vi "Upgrade Addon to Latest Version.vi"(8 "error in (no error)":errorcluster, 11 "Device Item Ref in in":T1 format="%.0x") -> (0 "error out":errorcluster, 3 "Device Item Ref out":T1 format="%.0x")   [LabVIEW 2026, in "FPGA Addon Shared.lvlib"]
uses:
  FPGA Addon Shared.lvlib
  <vilib>/NI VeriStand/Custom Device API/Custom Device Item Ref.ctl
  Types/FG Action.ctl
  Types/Register Information.ctl
  Types/FPGA Addon Data Type.ctl
  <vilib>/rvi/FIFO/Fifo_Types/Fifo_DMA_Config.ctl
  <vilib>/rvi/DataTransferAndStorage/Container/Common/niFpgaDataTypeControl.ctl
  <vilib>/rvi/ClientSDK/Core/ModuleGeneration/CommunicationInterfaceUtility/niFpgaDmaChannelImplementation.ctl
  Types/DMA Information.ctl
  Constants.vi
  <vilib>/NI/NI VeriStand Advanced SysDef API/_SubVIs/SysDef.Search.GUID.vi
  <vilib>/NI/NI VeriStand Advanced SysDef API/_SubVIs/SysDef.Property.Get.Variant.vi
  <vilib>/NI/NI VeriStand Advanced SysDef API/SysDef API/SysDef.Property.Set.vi
  <vilib>/NI/NI VeriStand Advanced SysDef API/_SubVIs/SysDef.Property.Set.Variant.vi
  <vilib>/NI/NI VeriStand Advanced SysDef API/_SubVIs/SysDef.Search.GUIDs.vi
  C:/Users/Administrator/Desktop/Jatin/All DNC DLLs/NationalInstruments.VeriStand.SystemDefinitionAPI.dll
  Jatin/All DNC DLLs/NationalInstruments.VeriStand.SystemDefinitionAPI.dll
  <vilib>/NI/NI VeriStand Advanced SysDef API/SysDef API/Advanced System Definition.lvlib
  <vilib>/NI VeriStand/Custom Device API/Custom Device API.lvlib
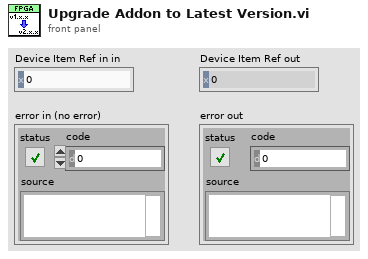
[diagram p1: front panel]
types:
  T1 = typedef "Custom Device API.lvlib/Custom Device Item Ref.ctl" = u64
  T2 = typedef "FPGA Addon Shared.lvlib/FG Action.ctl" = enum8{"GET", "SET"}
  T3 = typedef "FPGA Addon Shared.lvlib/Register Information.ctl" = cluster{"Name":string, "Data Type":T4, "Default Value":variant, "Attributes":variant}
  T4 = typedef "FPGA Addon Shared.lvlib/FPGA Addon Data Type.ctl" = enum8{"<Null>", "I8", "I16", "I32", "I64", "U8", "U16", "U32", "U64", "SGL", "Boolean", "Analog PWM In Settings", "Analog PWM In", "Digital PWM In Settings", "Digital PWM In", "Digital PWM Out", "Sine Out", "FXP", "FXP+/-24.5", "FXP+/-16.5", "FXP+/-32.8", "FXP+/-64.32", "FXP+/-16.7", "FXP+/-20.5", "FXP+/-27.5", "FXP+/-32.16", "FXP+16.3", "FXP+18.3", "Digital Static In", "Digital Static Out", "Digital Static In Settings", "Digital WSS Out", "Quad Encoder Settings", "Quad Encoder In", "Group"}
  T5 = typedef "FPGA Addon Shared.lvlib/DMA Information.ctl" = cluster{"Name":string, "Data Type":T4}
  T6 = cluster{"Name":string, "Data Type":enum8{"<Null>", "I8", "I16", "I32", "I64", "U8", "U16", "U32", "U64", "SGL", "Boolean", "Analog PWM In Settings", "Analog PWM In", "Digital PWM In Settings", "Digital PWM In", "Digital PWM Out", "Sine Out", "FXP+/-24.5", "FXP+/-16.5", "FXP+/-32.8", "FXP+/-64.32", "FXP+/-16.7", "FXP+/-20.5", "FXP+/-27.5", "FXP+/-32.16", "FXP+16.3", "FXP+18.3", "Digital Static In", "Digital Static Out", "Digital Static In Settings", "Digital WSS Out", "Quad Encoder Settings", "Quad Encoder In", "Group"}}[]
  T7 = cluster{"Name":string, "Data Type":enum8{"<Null>", "I8", "I16", "I32", "I64", "U8", "U16", "U32", "U64", "SGL", "Boolean", "Analog PWM In Settings", "Analog PWM In", "Digital PWM In Settings", "Digital PWM In", "Digital PWM Out", "Sine Out", "FXP+/-24.5", "FXP+/-16.5", "FXP+/-32.8", "FXP+/-64.32", "FXP+/-16.7", "FXP+/-20.5", "FXP+/-27.5", "FXP+/-32.16", "FXP+16.3", "FXP+18.3", "Digital Static In", "Digital Static Out", "Digital Static In Settings", "Digital WSS Out", "Quad Encoder Settings", "Quad Encoder In", "Group"}, "Default Value":variant}[]
  T8 = cluster{"Name":string, "Data Type":enum8{"<Null>", "I8", "I16", "I32", "I64", "U8", "U16", "U32", "U64", "SGL", "DBL", "EXT", "CSG", "CDB", "CXT", "0x0F", "0x10", "0x11", "0x12", "0x13", "0x14", "Enum U8", "Enum U16", "Enum U32", "Enum U64", "SGL PQ", "DBL PQ", "EXT PQ", "CSG PQ", "CDB PQ", "CXT PQ", "0x1F", "0x20", "Boolean", "0x22", "0x23", "0x24", "0x25", "0x26", "0x27", "0x28", "0x29", "0x2A", "0x2B", "0x2C", "0x2D", "0x2E", "0x2F", "String", "0x31", "Path", "Pict", "0x34", "0x35", "0x36", "DAQ", "0x38", "0x39", "0x3A", "0x3B", "0x3C", "0x3D", "0x3E", "0x3F", "Array", "0x41", "0x42", "0x43", "0x44", "0x45", "0x46", "0x47", "0x48", "0x49", "0x4A", "0x4B", "0x4C", "0x4D", "0x4E", "0x4F", "Cluster", "0x51", "0x52", "Variant", "Waveform", "0x55", "0x56", "0x57", "0x58", "0x59", "0x5A", "0x5B", "0x5C", "0x5D", "0x5E", "0x5F", "0x60", "0x61", "0x62", "0x63", "0x64", "0x65", "0x66", "0x67", "0x68", "0x69", "0x6A", "0x6B", "0x6C", "0x6D", "0x6E", "0x6F", "Refnum"}, "Default Value":dbl}[]
  T9 = enum8{"<Null>", "I8", "I16", "I32", "I64", "U8", "U16", "U32", "U64", "SGL", "DBL", "EXT", "CSG", "CDB", "CXT", "0x0F", "0x10", "0x11", "0x12", "0x13", "0x14", "Enum U8", "Enum U16", "Enum U32", "Enum U64", "SGL PQ", "DBL PQ", "EXT PQ", "CSG PQ", "CDB PQ", "CXT PQ", "0x1F", "0x20", "Boolean", "0x22", "0x23", "0x24", "0x25", "0x26", "0x27", "0x28", "0x29", "0x2A", "0x2B", "0x2C", "0x2D", "0x2E", "0x2F", "String", "0x31", "Path", "Pict", "0x34", "0x35", "0x36", "DAQ", "0x38", "0x39", "0x3A", "0x3B", "0x3C", "0x3D", "0x3E", "0x3F", "Array", "0x41", "0x42", "0x43", "0x44", "0x45", "0x46", "0x47", "0x48", "0x49", "0x4A", "0x4B", "0x4C", "0x4D", "0x4E", "0x4F", "Cluster", "0x51", "0x52", "Variant", "Waveform", "0x55", "0x56", "0x57", "0x58", "0x59", "0x5A", "0x5B", "0x5C", "0x5D", "0x5E", "0x5F", "0x60", "0x61", "0x62", "0x63", "0x64", "0x65", "0x66", "0x67", "0x68", "0x69", "0x6A", "0x6B", "0x6C", "0x6D", "0x6E", "0x6F", "Refnum"}
  T10 = typedef "Fifo_DMA_Config.ctl" = cluster{"Name":string, "Depth":u32, "Write? (Deprecated:Use Implementation)":bool, "Physical Channel":u32, "Base Address":u32, "Data Width":u32, "Data Type":T11, "FXP Properties":variant, "Write Window Address":u32, "Implementation":T12, "Control Set":u32}
  T11 = typedef "niFpgaDataTypeControl.ctl" = enum32{"Boolean", "I8", "I16", "I32", "I64", "U8", "U16", "U32", "U64", "FXP", "CustomControl", "SGL"}
  T12 = typedef "niFpgaDmaChannelImplementation.ctl" = enum16{"niFpgaTargetToHost", "niFpgaHostToTarget", "niFpgaPeerToPeerWriter", "niFpgaPeerToPeerReader", "niCoreTargetToHost", "niCoreHostToTarget", "niMemoryBufferReader", "niMemoryBufferWriter"}
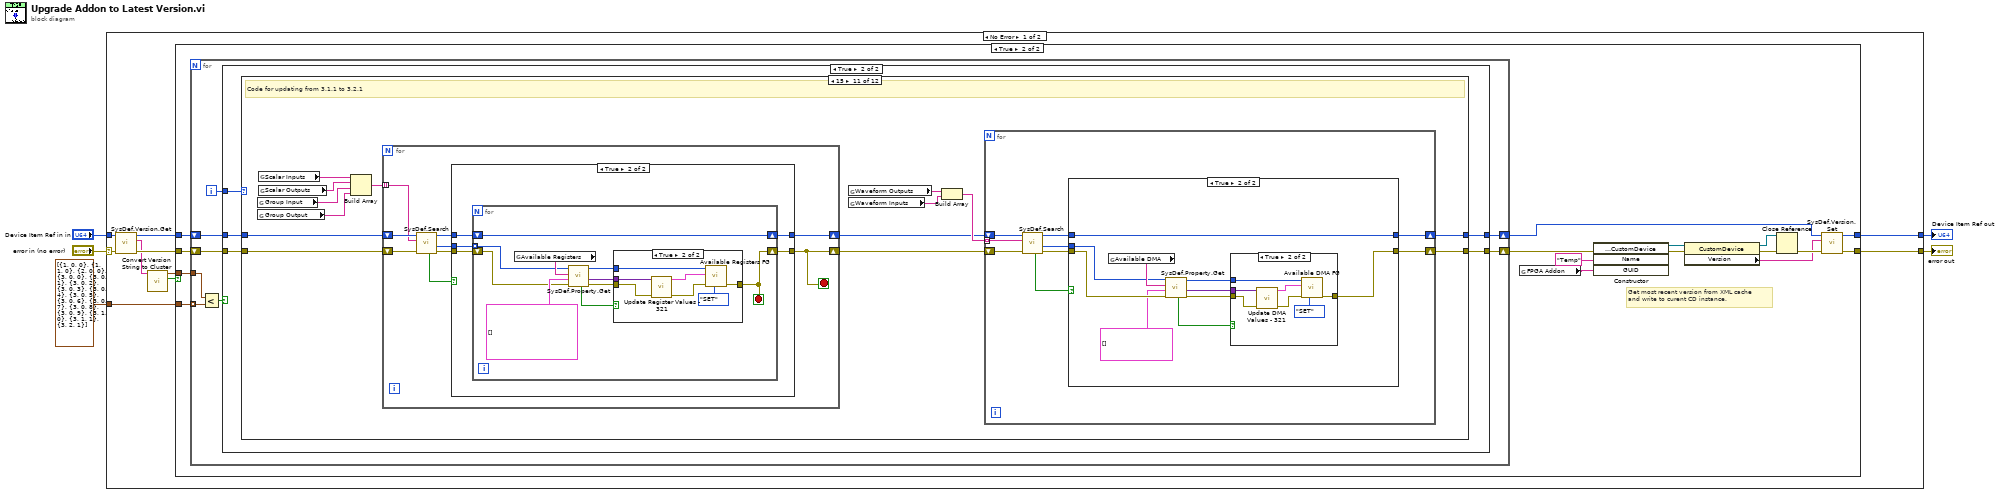
[diagram p0: block diagram]
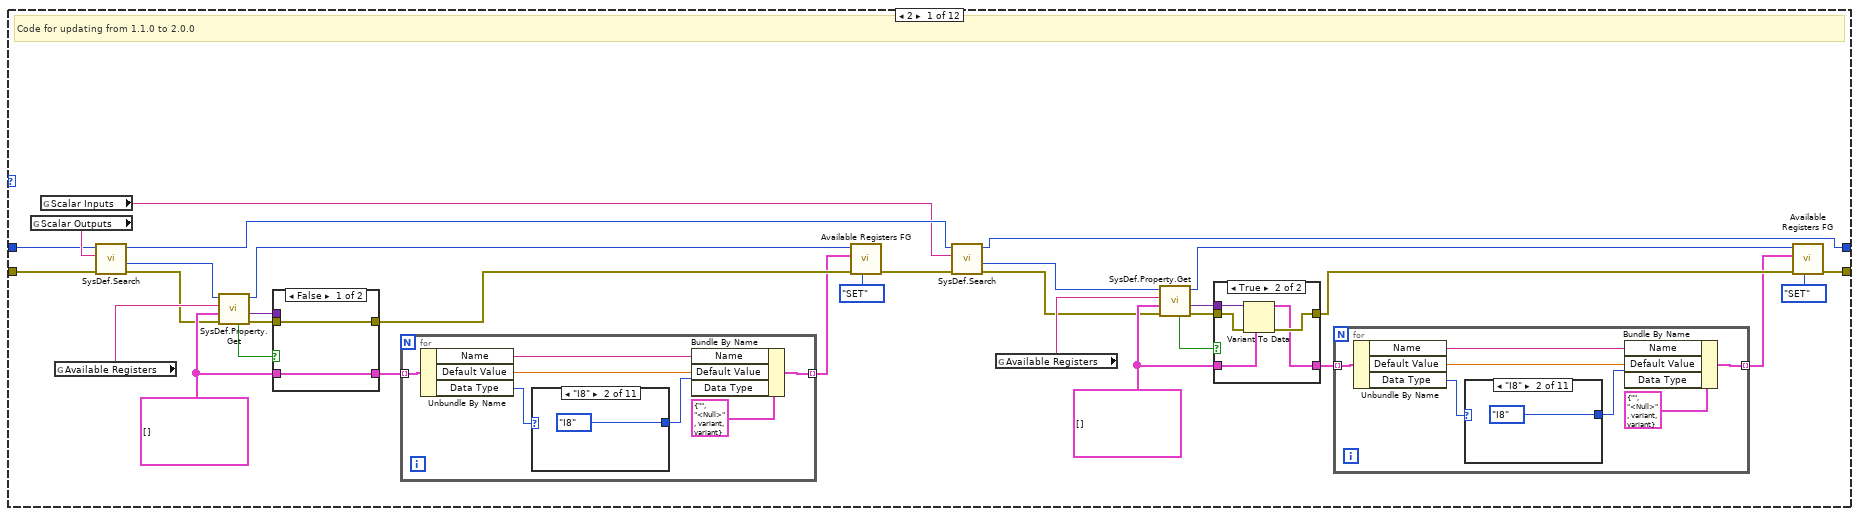
[diagram p4: hidden frame]
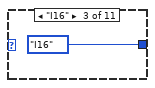
[diagram p6: hidden frame]
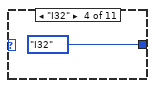
[diagram p7: hidden frame]
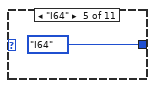
[diagram p8: hidden frame]
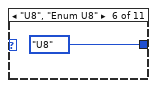
[diagram p9: hidden frame]
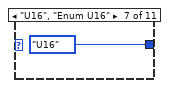
[diagram p10: hidden frame]
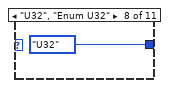
[diagram p11: hidden frame]
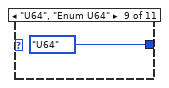
[diagram p12: hidden frame]
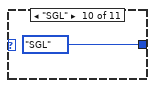
[diagram p13: hidden frame]
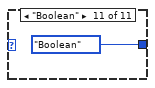
[diagram p14: hidden frame]
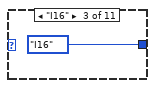
[diagram p17: hidden frame]
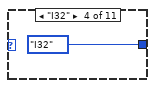
[diagram p18: hidden frame]
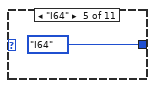
[diagram p19: hidden frame]
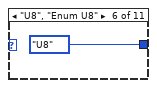
[diagram p20: hidden frame]
diagram:
  n1 = case shown="No Error" "error in (no error)" {
    selector: "error in (no error)" -> [w13 w290]
    tunnel: [w15 w290] -> w4
    tunnel: "Device Item Ref in in" -> [w12 w289]
    tunnel: [w14 w289] -> w5
    tunnel: cluster{i32, i32, i32}[] [{1, 0, 0}, {1, 1, 0}, {2, 0, 0}, {3, 0, 0}, {3, 0, 1}, {3, 0, 2}, {3, 0, 3}, {3, 0, 4}, {3, 0, 5}, {3, 0, 6}, {3, 0, 7}, {3, 0, 8}, {3, 0, 9}, {3, 1, 0}, {3, 1, 1}, {3, 2, 1}] -> [w9 _]
    frame No Error {
      n2 = call <vilib>:"SysDef.Version.Get.vi"("error in (no error)"=w13, "nodeID"=w12) -> ("error out"=w10:errorcluster, "Version"=w8:string, "nodeID out"=w11:u64)  [unwired: 7 in]
      n3 = call "Convert Version String to Cluster.vi"("Version"=w8) -> ("Version Valid?"=w6:bool, "Version"=w7:cluster{i32, i32, i32})  [unwired: 9 in]
      n4 = case shown="True" w6 {
        tunnel: [w17 w27] -> w15
        tunnel: [w16 w26] -> w14
        tunnel: w11 -> [w16 w21]
        tunnel: w10 -> [w17 w20]
        tunnel: w9 -> [_ w19]
        tunnel: w7 -> [_ w18]
        frame False {
        }
        frame True {
          # "Get most recent version from XML cache\nand write to curent CD instance."
          n5 = for {
            shift-right: [w41] -> w24
            shift-left: w20 -> [w34]
            shift-right: [w40] -> w25
            shift-left: w21 -> [w35]
            tunnel: w18 -> [w38]
            tunnel: w19 -> [w36] mode=indexing
            i -> [w39]
            n6 = Less?(x=w38, y=w36) -> (x < y?=w37:bool)
            n7 = case shown="True" w37 {
              tunnel: w34 -> [w43 w48]
              tunnel: [w43 w47] -> w41
              tunnel: w35 -> [w42 w44]
              tunnel: [w42 w45] -> w40
              tunnel: w39 -> [_ w46]
              frame False {
              }
              frame True {
                n8 = case shown="15" w46 {
                  tunnel: w48 -> [w74 w154 w186 w188 w190 w192 w194 w201 w207 w209 w223 w288]
                  tunnel: [w49 w130 w186 w188 w190 w192 w194 w196 w207 w209 w210 w288] -> w47
                  tunnel: [w50 w131 w185 w187 w189 w191 w193 w195 w206 w208 w211 w287] -> w45
                  tunnel: w44 -> [w73 w153 w185 w187 w189 w191 w193 w200 w206 w208 w222 w287]
                  frame 2 {
                    w57 = T8 [] ("Available Registers 2")
                    w68 = T8 [] ("Available Registers 2")
                    # "Code for updating from 1.1.0 to 2.0.0"
                    n9 = global read "Constants.vi" "Scalar Outputs"() -> (w79:string)
                    n10 = global read "Constants.vi" "Scalar Inputs"() -> (w75:string)
                    n11 = global read "Constants.vi" "Available Registers"() -> (w69:string)
                    n12 = call-poly <vilib>:"SysDef.Search.vi"("error in (no error)"=w74, "GUID"=w79, "nodeID"=w73) -> ("error out"=w65:errorcluster, "Value out"=w67:u64, "nodeID out"=w76:u64)  [unwired: 5 in, 1 out]
                    n13 = call-poly <vilib>:"SysDef.Property.Get.vi"("error in (no error)"=w65, "Value"=w68, "Property Name"=w69, "nodeID"=w67) -> ("error out"=w71:errorcluster, "Value"=w70:variant, "nodeID out"=w66:u64, "Found?"=w72:bool)  [unwired: 4 in]
                    n14 = case shown="False" w72 {
                      tunnel: w70 -> [_ w128]
                      tunnel: w68 -> [w122 w127]
                      tunnel: w71 -> [w123 w126]
                      tunnel: [w123 w125] -> w64
                      tunnel: [w122 w124] -> w63
                      frame False {
                      }
                      frame True {
                        n15 = Variant To Data(error in=w126, type=w127, Variant=w128) -> (data=w124:T8, error out=w125:errorcluster)
                      }
                    }
                    n16 = for {
                      tunnel: w63 -> [w111] mode=indexing
                      tunnel: [w107] -> w62 mode=indexing
                      n17 = Unbundle By Name(w111) -> ("Name"=w110:string, "Default Value"=w109:dbl, "Data Type"=w106:T9)
                      n18 = case shown="\"I8\"" w106 {
                        tunnel: [_ FPGA_Addon_Data_Type."I8" ("Data Type") FPGA_Addon_Data_Type."I16" ("Data Type") FPGA_Addon_Data_Type."I32" ("Data Type") FPGA_Addon_Data_Type."I64" ("Data Type") FPGA_Addon_Data_Type."U8" ("Data Type") FPGA_Addon_Data_Type."U16" ("Data Type") FPGA_Addon_Data_Type."U32" ("Data Type") FPGA_Addon_Data_Type."U64" ("Data Type") FPGA_Addon_Data_Type."SGL" ("Data Type") FPGA_Addon_Data_Type."Boolean" ("Data Type")] -> w105
                        frame Default {
                        }
                        frame "I8" {
                        }
                        frame "I16" {
                        }
                        frame "I32" {
                        }
                        frame "I64" {
                        }
                        frame "U8", "Enum U8" {
                        }
                        frame "U16", "Enum U16" {
                        }
                        frame "U32", "Enum U32" {
                        }
                        frame "U64", "Enum U64" {
                        }
                        frame "SGL" {
                        }
                        frame "Boolean" {
                        }
                      }
                      n19 = Bundle By Name(cluster=T3 {"Name"="", "Data Type"=enum."<Null>", "Default Value"=variant(refnum<class> refnum), "Attributes"=variant}, "Name"=w110, "Default Value"=w109, "Data Type"=w105) -> (w107:T3)
                    }
                    n20 = call "Available Registers FG.vi"("Action"=FG_Action."SET", "error in (no error)"=w64, "Available Registers"=w62, "Item Ref"=w66) -> ("error out"=w77:errorcluster)  [unwired: 5 in, 2 out]
                    n21 = call-poly <vilib>:"SysDef.Search.vi"("error in (no error)"=w77, "GUID"=w75, "nodeID"=w76) -> ("error out"=w55:errorcluster, "Value out"=w52:u64, "nodeID out"=w50:u64)  [unwired: 5 in, 1 out]
                    n22 = global read "Constants.vi" "Available Registers"() -> (w58:string)
                    n23 = call-poly <vilib>:"SysDef.Property.Get.vi"("error in (no error)"=w55, "Value"=w57, "Property Name"=w58, "nodeID"=w52) -> ("error out"=w60:errorcluster, "Value"=w59:variant, "nodeID out"=w51:u64, "Found?"=w61:bool)  [unwired: 4 in]
                    n24 = case shown="True" w61 {
                      tunnel: w59 -> [_ w104]
                      tunnel: w57 -> [w98 w103]
                      tunnel: w60 -> [w99 w102]
                      tunnel: [w99 w101] -> w54
                      tunnel: [w98 w100] -> w56
                      frame False {
                      }
                      frame True {
                        n25 = Variant To Data(error in=w102, type=w103, Variant=w104) -> (data=w100:T8, error out=w101:errorcluster)
                      }
                    }
                    n26 = for {
                      tunnel: w56 -> [w87] mode=indexing
                      tunnel: [w83] -> w53 mode=indexing
                      n27 = Unbundle By Name(w87) -> ("Name"=w86:string, "Default Value"=w85:dbl, "Data Type"=w82:T9)
                      n28 = case shown="\"I8\"" w82 {
                        tunnel: [_ FPGA_Addon_Data_Type."I8" ("Data Type") FPGA_Addon_Data_Type."I16" ("Data Type") FPGA_Addon_Data_Type."I32" ("Data Type") FPGA_Addon_Data_Type."I64" ("Data Type") FPGA_Addon_Data_Type."U8" ("Data Type") FPGA_Addon_Data_Type."U16" ("Data Type") FPGA_Addon_Data_Type."U32" ("Data Type") FPGA_Addon_Data_Type."U64" ("Data Type") FPGA_Addon_Data_Type."SGL" ("Data Type") FPGA_Addon_Data_Type."Boolean" ("Data Type")] -> w81
                        frame Default {
                        }
                        frame "I8" {
                        }
                        frame "I16" {
                        }
                        frame "I32" {
                        }
                        frame "I64" {
                        }
                        frame "U8", "Enum U8" {
                        }
                        frame "U16", "Enum U16" {
                        }
                        frame "U32", "Enum U32" {
                        }
                        frame "U64", "Enum U64" {
                        }
                        frame "SGL" {
                        }
                        frame "Boolean" {
                        }
                      }
                      n29 = Bundle By Name(cluster=T3 {"Name"="", "Data Type"=enum."<Null>", "Default Value"=variant(refnum<class> refnum), "Attributes"=variant}, "Name"=w86, "Default Value"=w85, "Data Type"=w81) -> (w83:T3)
                    }
                    n30 = call "Available Registers FG.vi"("Action"=FG_Action."SET", "error in (no error)"=w54, "Available Registers"=w53, "Item Ref"=w51) -> ("error out"=w49:errorcluster)  [unwired: 5 in, 2 out]
                  }
                  frame 5 {
                    w129 = T10[] [] ("Available Registers 2")
                    w138 = T10[] [] ("Available Registers 2")
                    # "Code for updating from 3.0.1 to 3.0.2"
                    n31 = global read "Constants.vi" "Waveform Outputs"() -> (w155:string)
                    n32 = global read "Constants.vi" "Waveform Inputs"() -> (w159:string)
                    n33 = global read "Constants.vi" "Available DMA"() -> (w149:string)
                    n34 = call-poly <vilib>:"SysDef.Search.vi"("error in (no error)"=w154, "GUID"=w159, "nodeID"=w153) -> ("error out"=w146:errorcluster, "Value out"=w148:u64, "nodeID out"=w156:u64)  [unwired: 5 in, 1 out]
                    n35 = call-poly <vilib>:"SysDef.Property.Get.vi"("error in (no error)"=w146, "Value"=w129, "Property Name"=w149, "nodeID"=w148) -> ("error out"=w151:errorcluster, "Value"=w150:variant, "nodeID out"=w147:u64, "Found?"=w152:bool)  [unwired: 4 in]
                    n36 = case shown="False" w152 {
                      tunnel: w150 -> [_ w184]
                      tunnel: w129 -> [w178 w183]
                      tunnel: w151 -> [w179 w182]
                      tunnel: [w179 w181] -> w145
                      tunnel: [w178 w180] -> w144
                      frame False {
                      }
                      frame True {
                        n37 = Variant To Data(error in=w182, type=w183, Variant=w184) -> (data=w180:T10[], error out=w181:errorcluster)
                      }
                    }
                    n38 = for {
                      tunnel: w144 -> [w177] mode=indexing
                      tunnel: [w175] -> w143 mode=indexing
                      n39 = Unbundle By Name(w177) -> ("Name"=w176:string)
                      n40 = Bundle By Name(cluster=T5 {"Name"="", "Data Type"=enum."<Null>"} ("Cluster"), "Name"=w176, "Data Type"=FPGA_Addon_Data_Type."SGL") -> (w175:T5)
                    }
                    n41 = call "Available DMA FG.vi"("Action"=FG_Action."SET", "error in (no error)"=w145, "Available DMA"=w143, "Item Ref"=w147) -> ("error out"=w157:errorcluster)  [unwired: 5 in, 2 out]
                    n42 = call-poly <vilib>:"SysDef.Search.vi"("error in (no error)"=w157, "GUID"=w155, "nodeID"=w156) -> ("error out"=w136:errorcluster, "Value out"=w133:u64, "nodeID out"=w131:u64)  [unwired: 5 in, 1 out]
                    n43 = global read "Constants.vi" "Available DMA"() -> (w139:string)
                    n44 = call-poly <vilib>:"SysDef.Property.Get.vi"("error in (no error)"=w136, "Value"=w138, "Property Name"=w139, "nodeID"=w133) -> ("error out"=w141:errorcluster, "Value"=w140:variant, "nodeID out"=w132:u64, "Found?"=w142:bool)  [unwired: 4 in]
                    n45 = case shown="False" w142 {
                      tunnel: w140 -> [_ w172]
                      tunnel: w138 -> [w166 w171]
                      tunnel: w141 -> [w167 w170]
                      tunnel: [w167 w169] -> w135
                      tunnel: [w166 w168] -> w137
                      frame False {
                      }
                      frame True {
                        n46 = Variant To Data(error in=w170, type=w171, Variant=w172) -> (data=w168:T10[], error out=w169:errorcluster)
                      }
                    }
                    n47 = for {
                      tunnel: w137 -> [w165] mode=indexing
                      tunnel: [w163] -> w134 mode=indexing
                      n48 = Unbundle By Name(w165) -> ("Name"=w164:string)
                      n49 = Bundle By Name(cluster=T5 {"Name"="", "Data Type"=enum."<Null>"} ("Cluster"), "Name"=w164, "Data Type"=FPGA_Addon_Data_Type."SGL") -> (w163:T5)
                    }
                    n50 = call "Available DMA FG.vi"("Action"=FG_Action."SET", "error in (no error)"=w135, "Available DMA"=w134, "Item Ref"=w132) -> ("error out"=w130:errorcluster)  [unwired: 5 in, 2 out]
                  }
                  frame 6 {
                    # "Code for updating from 3.0.2 to 3.0.3"
                  }
                  frame 7 {
                    # "Code for updating from 3.0.3 to 3.0.4"
                  }
                  frame 8 {
                    # "Code for updating from 3.0.4 to 3.0.5"
                  }
                  frame 9 {
                    # "Code for updating from 3.0.5 to 3.0.6"
                  }
                  frame 10 {
                    # "Code for updating from 3.0.6 to 3.0.7"
                  }
                  frame 11 {
                    # "Code for updating from 3.0.8 to 3.0.9"
                    n51 = global read "Constants.vi" "DMA Error"() -> (w199:string)
                    n52 = call-poly <vilib>:"SysDef.Search.vi"("error in (no error)"=w201, "GUID"=w199, "nodeID"=w200) -> ("error out"=w197:errorcluster, "Values Out"=w198:u64[], "nodeID out"=w195:u64)  [unwired: 5 in, 1 out]
                    n53 = for {
                      tunnel: w198 -> [w204] mode=indexing
                      shift-right: [w202] -> w196
                      shift-left: w197 -> [w205]
                      n54 = call <vilib>:"SysDef.Rename.vi"("error in (no error)"=w205, "Name"="Error Code", "nodeID"=w204) -> ("error out"=w202:errorcluster)  [unwired: 6 in, 2 out]
                    }
                  }
                  frame 12 {
                    # "Code for updating from 3.0.9 to 3.1.0"
                  }
                  frame 13 {
                    # "Code for updating from 3.1.0 to 3.1.1"
                  }
                  frame 15 {
                    # "Code for updating from 3.1.1 to 3.2.1"
                    n55 = global read "Constants.vi" "Group Input"() -> (w219:string)
                    n56 = global read "Constants.vi" "Group Output"() -> (w218:string)
                    n57 = global read "Constants.vi" "Scalar Inputs"() -> (w221:string)
                    n58 = global read "Constants.vi" "Scalar Outputs"() -> (w220:string)
                    n59 = Build Array(w221, w220, w219, w218) -> (w217:string[])
                    n60 = for {
                      tunnel: w217 -> [w258] mode=indexing
                      shift-right: [w253] -> w212
                      shift-left: w222 -> [w259]
                      shift-right: [w261] -> w213
                      shift-left: w223 -> [w260]
                      stop <- w261 stop-if-true
                      n61 = call-poly <vilib>:"SysDef.Search.vi"("error in (no error)"=w260, "GUID"=w258, "nodeID"=w259) -> ("error out"=w256:errorcluster, "Values Out"=w254:u64[], "nodeID out"=w255:u64, "Found?"=w257:bool)  [unwired: 5 in]
                      n62 = case shown="True" w257 {
                        tunnel: [w262 w268] -> w261
                        tunnel: w256 -> [w262 w266]
                        tunnel: w255 -> [w263 w265]
                        tunnel: w254 -> [_ w267]
                        tunnel: [w263 w264] -> w253
                        frame False {
                        }
                        frame True {
                          n63 = for {
                            tunnel: w267 -> [w272] mode=indexing
                            shift-right: [w270] -> w264
                            shift-left: w265 -> [w270]
                            shift-right: [w269] -> w268
                            shift-left: w266 -> [w271]
                            stop <- w269 stop-if-true
                            n64 = global read "Constants.vi" "Available Registers"() -> (w278:string)
                            n65 = call-poly <vilib>:"SysDef.Property.Get.vi"("error in (no error)"=w271, "Value"=T7 [] ("Available Registers 2"), "Property Name"=w278, "nodeID"=w272) -> ("error out"=w275:errorcluster, "Value"=w276:variant, "nodeID out"=w274:u64, "Found?"=w273:bool)  [unwired: 4 in]
                            n66 = case shown="True" w273 {
                              tunnel: w276 -> [_ w286]
                              tunnel: w275 -> [w279 w285]
                              tunnel: w274 -> [_ w281]
                              tunnel: [w279 w280] -> w269
                              frame False {
                              }
                              frame True {
                                n67 = call "Update Register Values - 321.vi"("error in (no error)"=w285, "Register Value"=w286) -> ("error out"=w283:errorcluster, "Updated Register Values"=w282:T3[])  [unwired: 8 in]
                                n68 = call "Available Registers FG.vi"("Action"=FG_Action."SET", "error in (no error)"=w283, "Available Registers"=w282, "Item Ref"=w281) -> ("error out"=w280:errorcluster)  [unwired: 5 in, 2 out]
                              }
                            }
                          }
                        }
                      }
                    }
                    n69 = global read "Constants.vi" "Waveform Outputs"() -> (w216:string)
                    n70 = global read "Constants.vi" "Waveform Inputs"() -> (w215:string)
                    n71 = Build Array(w216, w215) -> (w214:string[])
                    n72 = for {
                      tunnel: w214 -> [w230] mode=indexing
                      shift-right: [w224] -> w210
                      shift-left: w213 -> [w232]
                      shift-right: [w225] -> w211
                      shift-left: w212 -> [w231]
                      n73 = call-poly <vilib>:"SysDef.Search.vi"("error in (no error)"=w232, "GUID"=w230, "nodeID"=w231) -> ("error out"=w229:errorcluster, "Value out"=w227:u64, "nodeID out"=w226:u64, "Found?"=w228:bool)  [unwired: 5 in]
                      n74 = case shown="True" w228 {
                        tunnel: w229 -> [w233 w244]
                        tunnel: w227 -> [_ w237]
                        tunnel: w226 -> [w234 w236]
                        tunnel: [w234 w236] -> w225
                        tunnel: [w233 w235] -> w224
                        frame False {
                        }
                        frame True {
                          n75 = global read "Constants.vi" "Available DMA"() -> (w243:string)
                          n76 = call-poly <vilib>:"SysDef.Property.Get.vi"("error in (no error)"=w244, "Value"=T6 [] ("Available DMA"), "Property Name"=w243, "nodeID"=w237) -> ("error out"=w239:errorcluster, "Value"=w240:variant, "nodeID out"=w238:u64, "Found?"=w241:bool)  [unwired: 4 in]
                          n77 = case shown="True" w241 {
                            tunnel: w240 -> [_ w251]
                            tunnel: w239 -> [w245 w252]
                            tunnel: w238 -> [_ w250]
                            tunnel: [w245 w246] -> w235
                            frame False {
                            }
                            frame True {
                              n78 = call "Update DMA Values - 321.vi"("error in (no error)"=w252, "Register Value"=w251) -> ("error out"=w248:errorcluster, "Updated DMA Values"=w249:T5[])  [unwired: 8 in]
                              n79 = call "Available DMA FG.vi"("Action"=FG_Action."SET", "error in (no error)"=w248, "Available DMA"=w249, "Item Ref"=w250) -> ("error out"=w246:errorcluster)  [unwired: 5 in, 2 out]
                            }
                          }
                        }
                      }
                    }
                  }
                  frame Default {
                  }
                }
              }
            }
          }
          n80 = global read "Constants.vi" "FPGA Addon"() -> (w22:string)
          n81 = constructor class="CustomDevice"(error in=w24, "Name"="Temp", "GUID"=w22) -> (reference out=w33:refnum<k39>, error out=w32:errorcluster)  [unwired: 2 in, 3 out]
          n82 = property class="CustomDevice"(reference=w33, error in=w32) -> (reference out=w30:refnum<k39>, error out=w31:errorcluster, "Version"=w28:string)
          n83 = Close Reference(reference=w30, error in (no error)=w31) -> (error out=w29:errorcluster)
          n84 = call <vilib>:"SysDef.Version.Set.vi"("error in (no error)"=w29, "Version"=w28, "nodeID"=w25) -> ("error out"=w27:errorcluster, "nodeID out"=w26:u64)  [unwired: 7 in]
        }
      }
    }
    frame Error {
    }
  }
  "Device Item Ref out" <- w5
  "error out" <- w4
